vi "write remote chassis.vi"(8 "error in":errorcluster, 10 "remote chassis":refnum<class "Chassis.lvclass">[](array[class]), 11 "Controller in":refnum<class "Controller.lvclass">) -> (0 "error out":errorcluster, 3 "Controller out":refnum<class "Controller.lvclass">)   [LabVIEW 2016, in "SMI.lvlib" / "Controller.lvclass"]
uses:
  Controller.lvclass
  Chassis/Chassis.lvclass
  Controller.lvclass/Controller.ctl
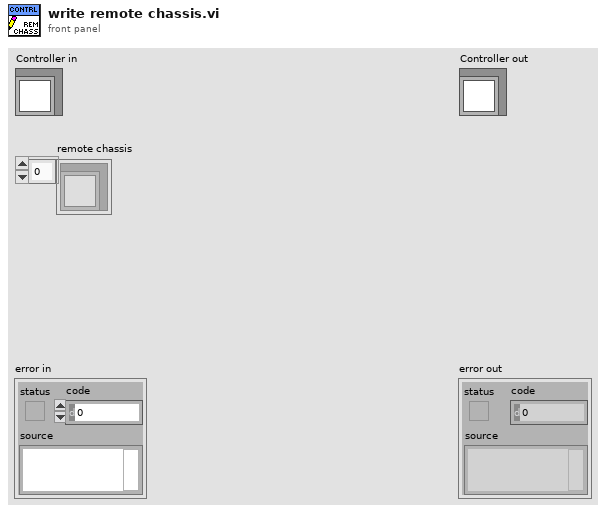
[diagram p1: front panel]
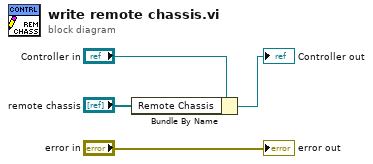
[diagram p0: block diagram]
diagram:
  n1 = Bundle By Name(cluster="Controller in", "Remote Chassis"="remote chassis") -> (→"Controller out":refnum<class "Controller.lvclass">)
  "error out" <- "error in"
